vi "column count.vi"(8 "error in (no error)":errorcluster, 11 "SQLite3LV Cursor in":refnum<class "cursor.lvclass">) -> (0 "error out":errorcluster, 2 "# of columns":i32, 3 "SQLite3LV Cursor out":refnum<class "cursor.lvclass">)   [LabVIEW 2014, in "SQLite3LV.lvlib" / "cursor.lvclass"]
uses:
  cursor.lvclass
  cursor.lvclass/cursor.ctl
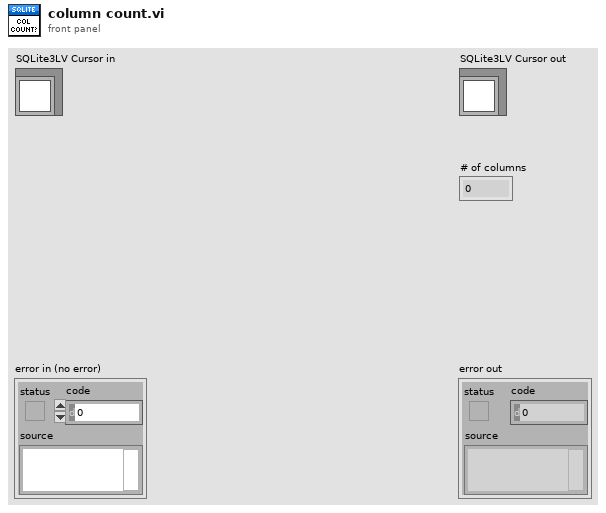
[diagram p1: front panel]
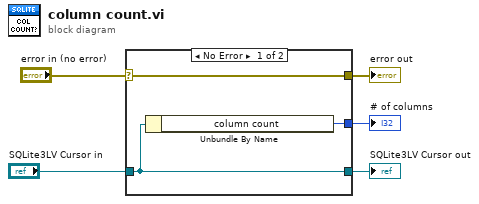
[diagram p0: block diagram]
diagram:
  n1 = case shown="No Error" "error in (no error)" {
    selector: "error in (no error)" -> [w8 w10]
    tunnel: [w8 w10] -> w5
    tunnel: [w7 w9] -> w4
    tunnel: "SQLite3LV Cursor in" -> [w7 w9]
    tunnel: [w6 _] -> w3
    frame No Error {
      n2 = Unbundle By Name(w7) -> ("column count"=w6:i32)
    }
    frame Error {
    }
  }
  "error out" <- w5
  "SQLite3LV Cursor out" <- w4
  "# of columns" <- w3
